vi "Read TSF MNGR.vi"(8 "error in (no error)":errorcluster, 11 "QPA Measurement in":refnum<class "QPA Measurement.lvclass">=refnum) -> (0 "error out":errorcluster, 2 "TSF Parser.lvlibp:TSF Parser.lvclass":refnum<class "TSF Parser.lvclass">, 3 "QPA Measurement out":refnum<class "QPA Measurement.lvclass">)   [LabVIEW 2016, in "QPA Measurement.lvlib" / "QPA Measurement.lvclass"]
uses:
  QPA Measurement.lvclass
  Plugins/TSF Parser.lvlibp/TSF Parser.lvclass
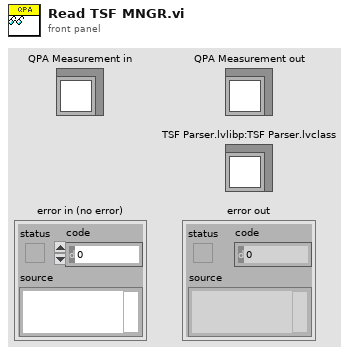
[diagram p1: front panel]
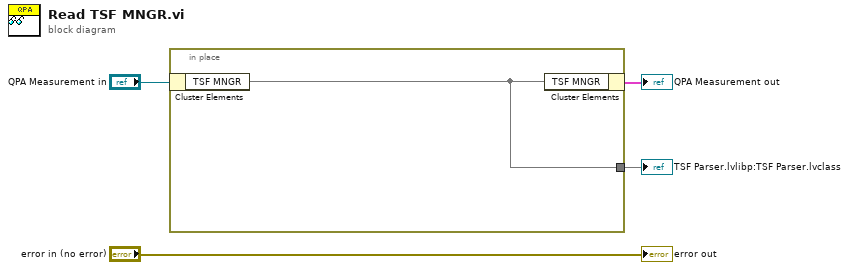
[diagram p0: block diagram]
diagram:
  n1 = in-place {
    in-place-border: [w5] -> w2
    n2 = in-place-cluster #1("QPA Measurement in") -> ("TSF MNGR"=w5)
    n3 = in-place-cluster #1("TSF MNGR"=w5) -> (→"QPA Measurement out":cluster{})
  }
  "TSF Parser.lvlibp:TSF Parser.lvclass" <- w2
  "error out" <- "error in (no error)"
